vi "List Children Priv.vi"(0 "Tree Dictionary":variant, 7 "Parent ID":string, 11 "Error In":errorcluster) -> (4 "Tree Dictionary Out":variant, 8 "Child IDs":string[](array[string]), 15 "Error Out":errorcluster)   [LabVIEW 2020, in "NI_VIAnCFGDataStructure.lvlib" / "Tree.lvclass"]
uses:
  <vilib>/addons/analyzer/VIAnCFGDataStructure/Tree Manager/Tree.lvclass
  <vilib>/addons/analyzer/VIAnCFGDataStructure/Tree Manager/Typedefs/Tree Cluster.ctl
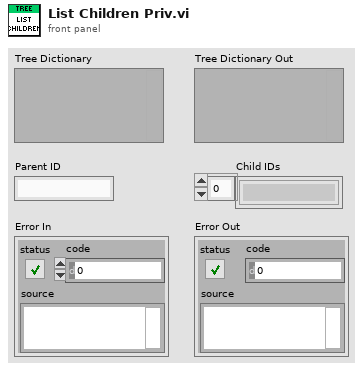
[diagram p1: front panel]
types:
  T1 = typedef "NI_VIAnCFGDataStructure.lvlib/Tree.lvclass/Tree Cluster.ctl" = cluster{"Unique ID":string, "Parent ID":string, "Child IDs":string[], "Name":string, "MetaData":string, "Data IDs":string[]}
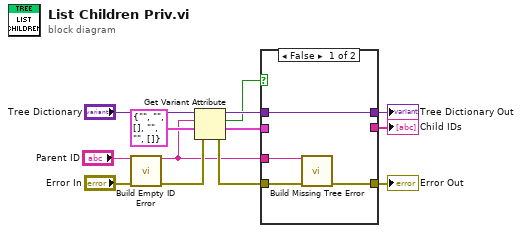
[diagram p0: block diagram]
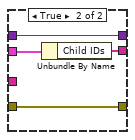
[diagram p2: hidden frame]
diagram:
  n1 = call <vilib>:"Build Empty ID Error.vi"("Unique ID"="Parent ID", "Error In"="Error In") -> ("Unique ID Out"=w1:string, "Error Out"=w3:errorcluster)  [unwired: 12 in]
  n2 = Get Variant Attribute(Variant="Tree Dictionary", name=w1, default value (empty Variant)=T1 {"Unique ID"="", "Parent ID"="", "Child IDs"=[], "Name"="", "MetaData"="", "Data IDs"=[]} ("Cluster of class private data"), error in=w3) -> (duplicate Variant=w9:variant, found=w7:bool, value=w11:T1, error out=w13:errorcluster)
  n3 = case shown="False" w7 {
    tunnel: [w17 w19] -> w8
    tunnel: w9 -> [w17 w19]
    tunnel: w1 -> [w16 _]
    tunnel: [w15 w18] -> w10
    tunnel: w11 -> [_ w21]
    tunnel: [_ w20] -> w12
    tunnel: w13 -> [w14 w18]
    frame False {
      n4 = call <vilib>:"Build Missing Tree Error.vi"("Unique ID"=w16, "Error In"=w14) -> ("Error Out"=w15:errorcluster)  [unwired: 13 in]
    }
    frame True {
      n5 = Unbundle By Name(w21) -> ("Child IDs"=w20:string[])
    }
  }
  "Child IDs" <- w12
  "Error Out" <- w10
  "Tree Dictionary Out" <- w8
